vi "AO_mini_slopes2zern_batch.vi"() -> ()   [LabVIEW 2018]
uses:
  <userlib>/WaveKit.lib/Controls/HasoSlopes.lvclass
panel:
  in  "Folder In":path=path "D:/Data/20200718_monitorBead/WF_processed/WF_abeFree_p5x1_1_rename"
  in  "Num End":dbl=999.0
  in  "Num Start":dbl
  in  "Folder Out":path=path "D:/Data/20200718_monitorBead/WF_processed/WF_abeFree_p5x1_1_Coeffs"
  in  "Base Name":string="WF_"
  out "Zernike pupil":i32[][](graph)
  out "Measured pupil":i32[][](graph)
  out "Zernike Coefficients":sgl[](graph)
  out "error out":errorcluster
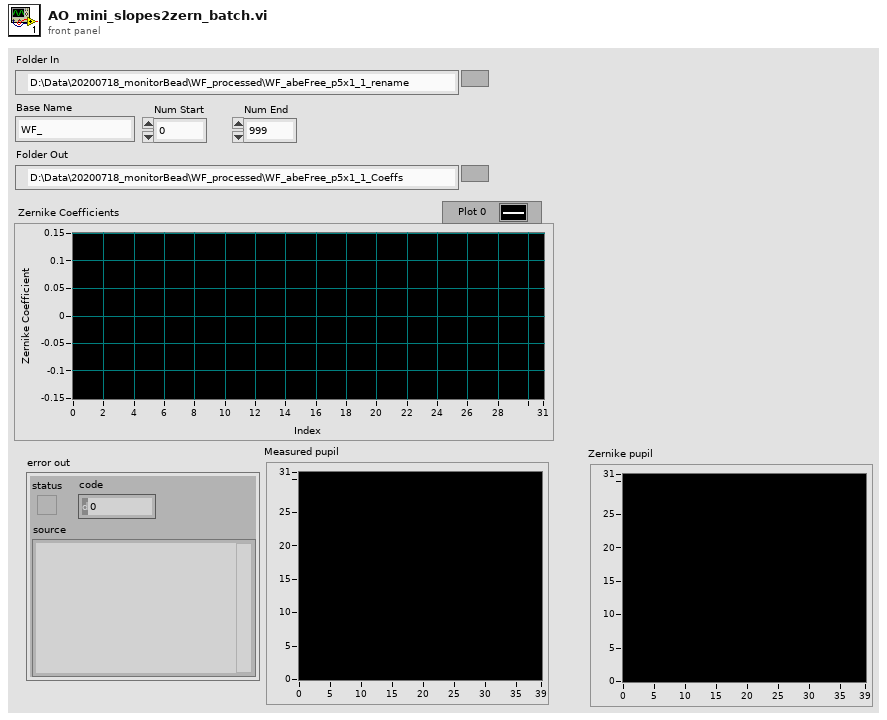
[diagram p1: front panel]
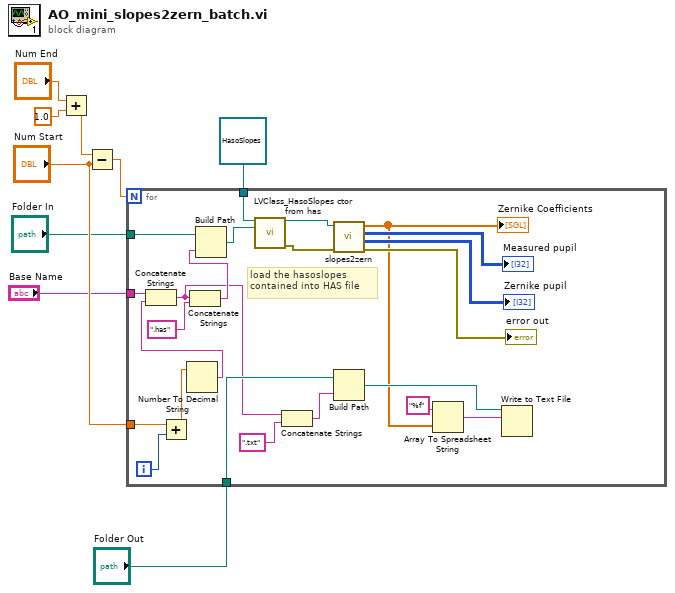
[diagram p0: block diagram]
diagram:
  n1 = Add(x="Num End", y=1.0) -> (x+y=w3:dbl)
  n2 = Subtract(x=w3, y="Num Start") -> (x-y=w7:dbl)
  n3 = for {
    N: w7 -> [_]
    tunnel: "Folder Out" -> [w27]
    tunnel: refnum<class "HasoSlopes.lvclass"> refnum ("HasoSlopes in") -> [w24]
    tunnel: "Num Start" -> [w20]
    tunnel: "Base Name" -> [w16]
    tunnel: "Folder In" -> [w13]
    i -> [w21]
    # "load the hasoslopes\ncontained into HAS file"
    n4 = Add(x=w20, y=w21) -> (x+y=w19:dbl)
    n5 = Number To Decimal String(number=w19) -> (decimal integer string=w17:string)  [unwired: 1 in]
    n6 = Concatenate Strings(w16, w17) -> (w11:string)
    n7 = Concatenate Strings(w11, ".has") -> (w14:string)
    n8 = Build Path(base path=w13, name or relative path=w14) -> (appended path=w12:path)
    n9 = call <userlib>:"LVClass_HasoSlopes ctor from has.vi"("HasoSlopes in"=w24, ".has path"=w12) -> ("HasoSlopes out"=w23:refnum<class "HasoSlopes.lvclass">, "error out"=w22:errorcluster)  [unwired: 12 in]
    n10 = Concatenate Strings(w11, ".txt") -> (w10:string)
    n11 = call "slopes2zern.vi"("HasoSlopes in"=w23, "error in (no error)"=w22) -> ("Zernike Coefficients"=w25:sgl[], "Measured pupil"=→"Measured pupil":i32[][], "Zernike pupil"=→"Zernike pupil":i32[][], "error out"=→"error out":errorcluster)  [unwired: 4 in, 1 out]
    "Zernike Coefficients" <- w25
    n12 = Build Path(base path=w27, name or relative path=w10) -> (appended path=w26:path)
    n13 = Array To Spreadsheet String(array=w25, 3:"%f") -> (spreadsheet string=w28:string)  [unwired: 1 in]
    n14 = Write to Text File(file (use dialog)=w26, text=w28) -> ()  [unwired: 2 in, 3 out]
  }
